vi "Save Data (Attach).vi"(0 "Filepath":path, 3 "Data":string[](array[string]), 7 "xlRefs":T1, 11 "Error In":errorcluster) -> (15 "Error Out":errorcluster)   [LabVIEW 2013]
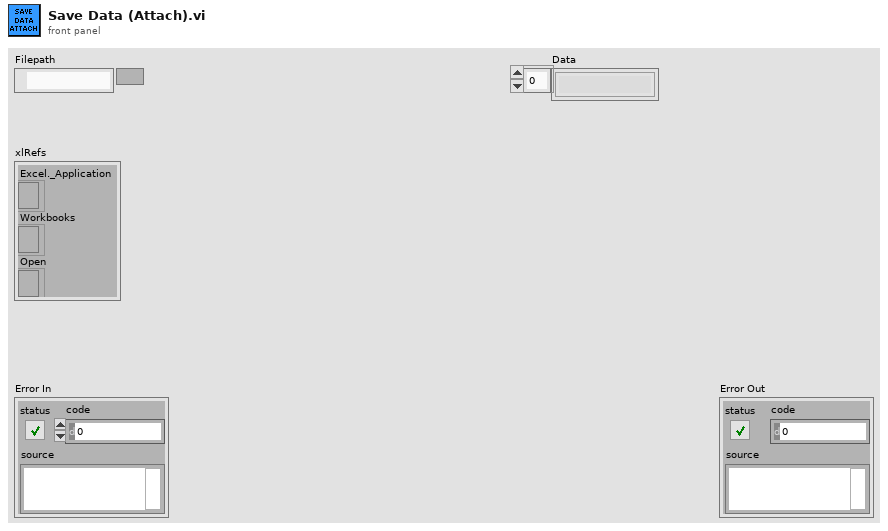
[diagram p1: front panel]
types:
  T1 = cluster{"Excel._Application":refnum<k7>, "Workbooks":refnum<k7>, "Open":refnum<k7>}
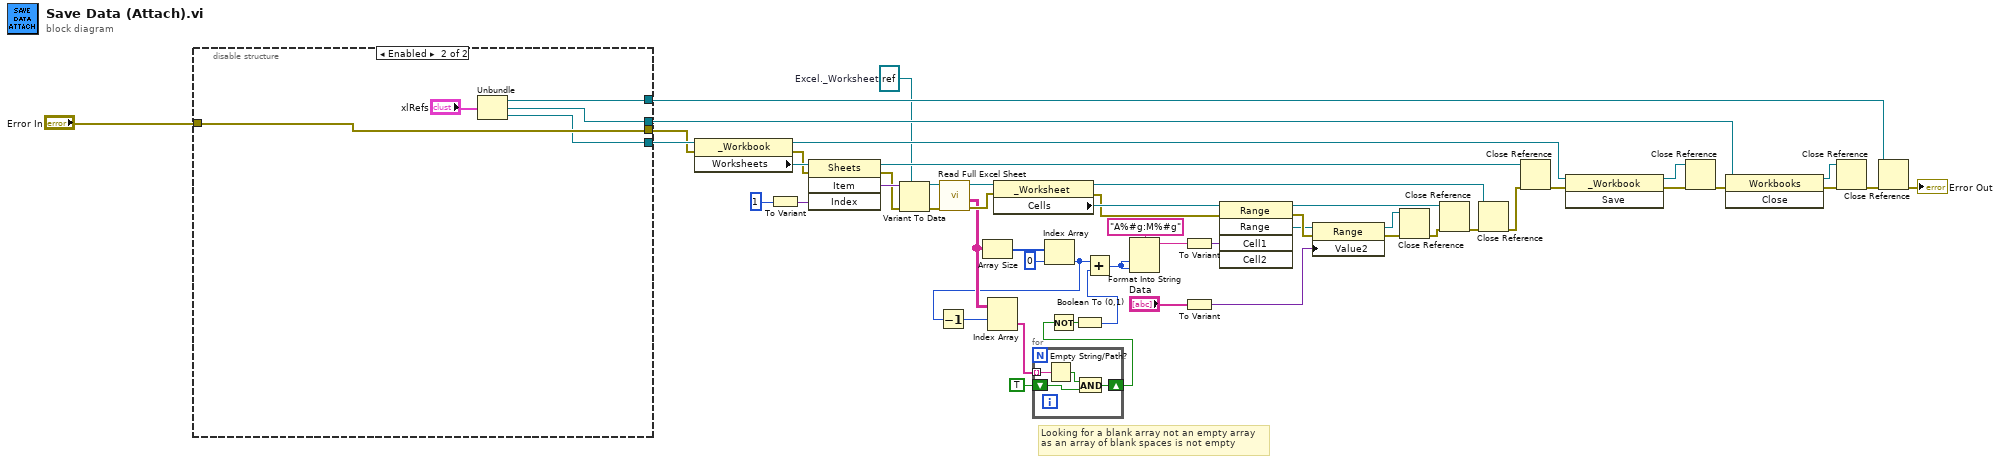
[diagram p0: block diagram]
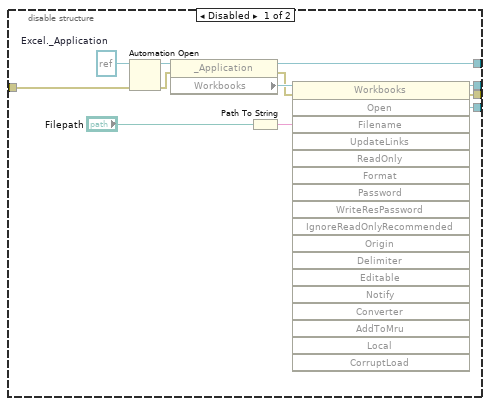
[diagram p2: hidden frame]
diagram:
  w39 = refnum<k7> refnum  # Excel._Worksheet
  # "Looking for a blank array not an empty array\nas an array of blank spaces is not empty"
  n1 = disable-structure shown="Enabled" {
    disable-tunnel: [w61 w66] -> w53
    disable-tunnel: [w60 w67] -> w51
    disable-tunnel: [w58 w68] -> w48
    disable-tunnel: [w57 w70] -> w47
    disable-tunnel: "Error In" -> [w55 w70]
    frame Disabled {
      w62 = refnum<k7> refnum  # Excel._Application
      n2 = Automation Open(error in (no error)=w55, Automation Refnum=w62) -> (Automation Refnum=w63:refnum<k7>, error out=w64:errorcluster)  [unwired: 2 in]
      n3 = property class="_Application"(reference=w63, error in=w64) -> (reference out=w58:refnum<k7>, error out=w59:errorcluster, "Workbooks"=w65:refnum<k7>)
      n4 = Path To String(path="Filepath") -> (string=w56:string)
      n5 = invoke class="Workbooks" method="Open"(reference=w65, error in=w59, "Filename"=w56) -> (reference out=w60:refnum<k7>, error out=w57:errorcluster, "Open"=w61:refnum<k7>)  [unwired: 15 in, 15 out]
    }
    frame Enabled {
      n6 = Unbundle("xlRefs") -> ("Excel._Application"=w68:refnum<k7>, "Workbooks"=w67:refnum<k7>, "Open"=w66:refnum<k7>)
    }
  }
  n7 = property class="_Workbook"(reference=w53, error in=w47) -> (reference out=w42:refnum<k7>, error out=w18:errorcluster, "Worksheets"=w19:refnum<k7>)
  n8 = To Variant(anything=1) -> (Variant=w34:variant)
  n9 = invoke class="Sheets" method="Item"(reference=w19, error in=w18, "Index"=w34) -> (reference out=w40:refnum<k7>, error out=w32:errorcluster, "Item"=w33:variant)  [unwired: 1 in, 1 out]
  n10 = Variant To Data(error in=w32, type=w39, Variant=w33) -> (data=w12:refnum<k7>, error out=w11:errorcluster)
  n11 = call "Read Full Excel Sheet.vi"("Error In"=w11, "Excel._Worksheet"=w12) -> ("Error Out"=w10:errorcluster, "Data"=w9:string[][], "Reference Out"=w13:refnum<k7>)  [unwired: 7 in]
  n12 = Array Size(array=w9) -> (size(s)=w17:i32[])
  n13 = property class="_Worksheet"(reference=w13, error in=w10) -> (reference out=w30:refnum<k7>, error out=w14:errorcluster, "Cells"=w15:refnum<k7>)
  n14 = Index Array(array=w17, index=0) -> (element=w5:i32)
  n15 = Decrement(x=w5) -> (x-1=w4:i32)
  n16 = Index Array(array=w9, index (row)=w4) -> (element=w3:string[])  [unwired: 1 in]
  n17 = for {
    tunnel: w3 -> [w74] mode=indexing
    shift-right: [w72] -> w1
    shift-left: TRUE -> [w71]
    n18 = Empty String/Path?(string/path=w74) -> (empty?=w73:bool)
    n19 = And(x=w73, y=w71) -> (x .and. y?=w72:bool)
  }
  n20 = Not(x=w1) -> (.not. x?=w8:bool)
  n21 = Boolean To (0,1)(Boolean=w8) -> (0, 1=w6:i16)
  n22 = Add(x=w5, y=w6) -> (x+y=w7:i32)
  n23 = Format Into String(format string="A%#g:M%#g", w7, w7) -> (resulting string=w21:string)  [unwired: 2 in, 1 out]
  n24 = To Variant(anything=w21) -> (Variant=w26:variant)
  n25 = To Variant(anything="Data") -> (Variant=w24:variant)
  n26 = invoke class="Range" method="Range"(reference=w15, error in=w14, "Cell1"=w26) -> (reference out=w29:refnum<k7>, error out=w25:errorcluster, "Range"=w20:refnum<k7>)  [unwired: 2 in, 2 out]
  n27 = property class="Range"(reference=w20, error in=w25, "Value2"=w24) -> (reference out=w23:refnum<k7>, error out=w22:errorcluster)
  n28 = Close Reference(reference=w23, error in (no error)=w22) -> (error out=w28:errorcluster)
  n29 = Close Reference(reference=w29, error in (no error)=w28) -> (error out=w31:errorcluster)
  n30 = Close Reference(reference=w30, error in (no error)=w31) -> (error out=w41:errorcluster)
  n31 = Close Reference(reference=w40, error in (no error)=w41) -> (error out=w46:errorcluster)
  n32 = invoke class="_Workbook" method="Save"(reference=w42, error in=w46) -> (reference out=w43:refnum<k7>, error out=w44:errorcluster)  [unwired: 1 in, 1 out]
  n33 = Close Reference(reference=w43, error in (no error)=w44) -> (error out=w45:errorcluster)
  n34 = invoke class="Workbooks" method="Close"(reference=w51, error in=w45) -> (reference out=w50:refnum<k7>, error out=w49:errorcluster)  [unwired: 1 in, 1 out]
  n35 = Close Reference(reference=w50, error in (no error)=w49) -> (error out=w52:errorcluster)
  n36 = Close Reference(reference=w48, error in (no error)=w52) -> (error out=→"Error Out":errorcluster)
